vi "CLSUIP_Generate Add Multiple Data Structure for Interface Tree.vi"(8 "error in":errorcluster, 10 "Interface Glyph Index":i32, 11 "Parent Interfaces":refnum<vi>[](array[refnum])) -> (0 "error out":errorcluster, 3 "Add Multiple Data Structure for Tree":T1(array[cluster]))   [LabVIEW 2021]
panel:
  in  "Missing Interface":string="This interface is missing.  Either it could not be found on disk, or an LabVIEW encountered an error trying to load it."
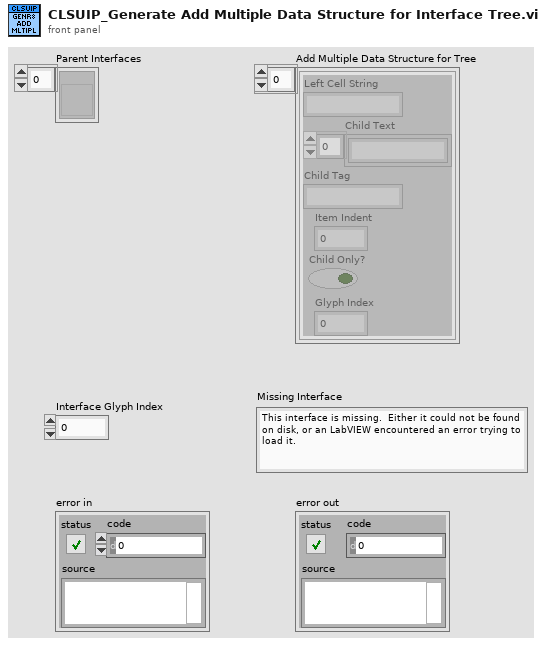
[diagram p1: front panel]
types:
  T1 = cluster{"Left Cell String":string, "Child Text":string[], "Child Tag":string, "Item Indent":i32, "Child Only?":bool, "Glyph Index":i32}[]
  T2 = cluster{"Left Cell String":string, "Child Text":string[], "Child Tag":string, "Item Indent":i32, "Child Only?":bool, "Glyph Index":i32}
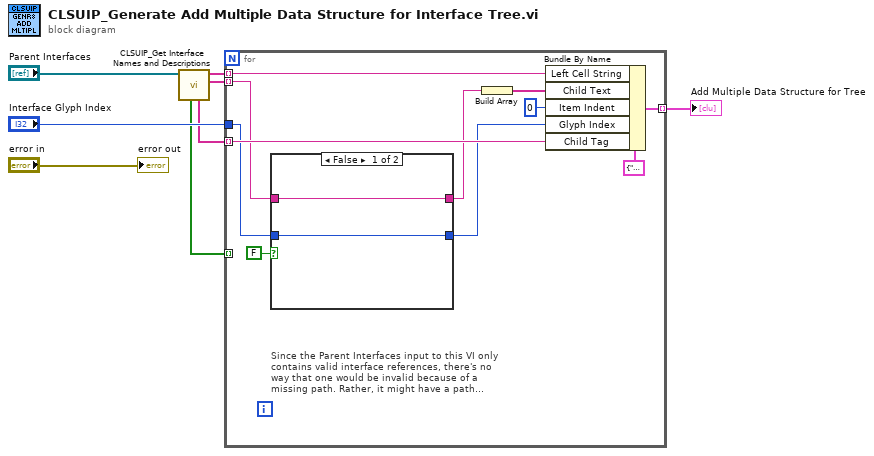
[diagram p0: block diagram]
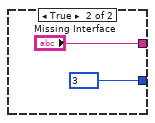
[diagram p2: hidden frame]
diagram:
  n1 = call <resource>:"CLSUIP_Get Interface Names and Descriptions.vi"("Interfaces"="Parent Interfaces") -> ("Descriptions"=w5:string[], "Qualified Names (without extensions)"=w6:string[], "Item IDs"=w2:string[], "Missing File"=w1:bool[])  [unwired: 6 in, 1 out]
  n2 = for {
    tunnel: w6 -> [w18] mode=indexing
    tunnel: w5 -> [w13] mode=indexing
    tunnel: "Interface Glyph Index" -> [w11]
    tunnel: [w15] -> w3 mode=indexing
    tunnel: w2 -> [w14] mode=indexing
    tunnel: w1 -> [_] mode=indexing
    n3 = case "Since the Parent Interfaces input to this VI only contains valid interface references, there's no way that one would be invalid because of a missing path. Rather, it might have a path assigned but not be saved to disk yet based on the late change in LV 2020 that assigned paths to unsaved classes and interfaces. So if we're to this point in this VI, we have a valid interface, it may or may not be saved to disk, and we don't need to check its status on disk to know it's valid. In summary, all interface references that come into this VI should be valid." shown="False" FALSE {
      tunnel: w13 -> [w21 _]
      tunnel: [w21 "Missing Interface"] -> w12
      tunnel: w11 -> [w20 _]
      tunnel: [w20 3] -> w10
      frame False {
      }
      frame True {
      }
    }
    n4 = Build Array(w12) -> (w17:string[])
    n5 = Bundle By Name(cluster=T2 {"Left Cell String"="", "Child Text"=[], "Child Tag"="", "Item Indent"=0, "Child Only?"=FALSE, "Glyph Index"=0} ("Item"), "Left Cell String"=w18, "Child Text"=w17, "Item Indent"=0, "Glyph Index"=w10, "Child Tag"=w14) -> (w15:T2)
  }
  "Add Multiple Data Structure for Tree" <- w3
  "error out" <- "error in"
